vi "Crosswalk.vi"() -> ()   [LabVIEW 2020]
uses:
  Auto.ctl
  People.ctl
  State.ctl
panel:
  out "Time Elapsed (s)":u32
  in  "Button":bool
  in  "stop":bool
  out "State":T1
  out "Pedestrians":T2
  out "Vehicles":T3
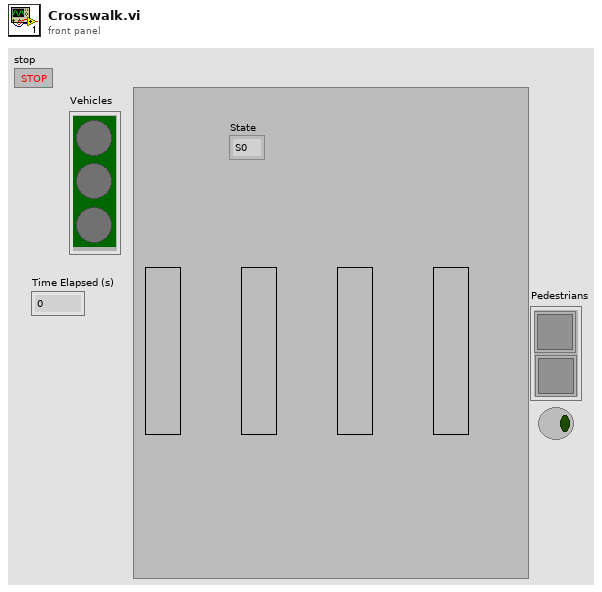
[diagram p1: front panel]
types:
  T1 = typedef "State.ctl" = enum16{"S0", "S1", "S2", "S3", "S4"}
  T2 = typedef "People.ctl" = cluster{"Red":bool, "Green":bool}
  T3 = typedef "Auto.ctl" = cluster{"Red":bool, "Yellow":bool, "Green":bool}
  T4 = enum8{"Enabled", "Disabled", "Disabled and Grayed Out"}
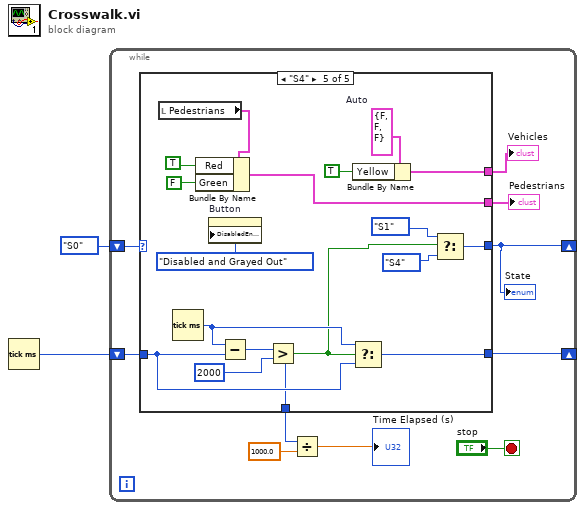
[diagram p0: block diagram]
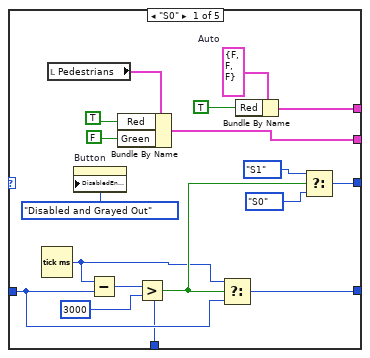
[diagram p2: hidden frame]
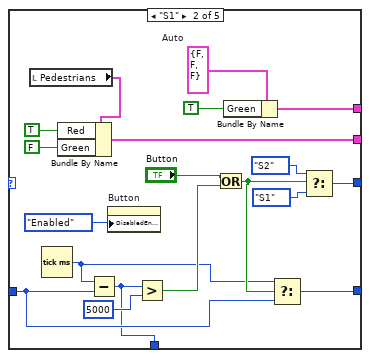
[diagram p3: hidden frame]
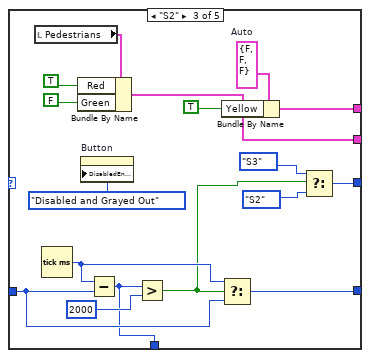
[diagram p4: hidden frame]
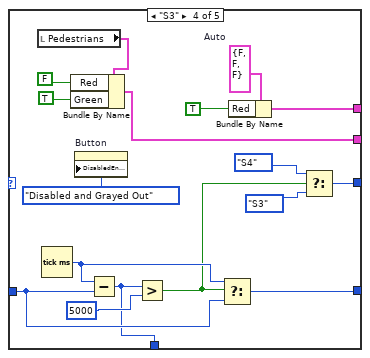
[diagram p5: hidden frame]
diagram:
  n1 = Tick Count (ms)() -> (millisecond timer value=w1:u32)
  n2 = while {
    shift-right: [w7] -> _
    shift-left: State."S0" ("Состояние") -> [w11]
    shift-right: [w10] -> _
    shift-left: w1 -> [w3]
    stop <- "stop" stop-if-true
    n3 = case shown="\"S4\"" w11 {
      tunnel: w3 -> [w27 w46 w62 w79 w96]
      tunnel: [w28 w47 w63 w80 w97] -> w10
      tunnel: [w24 w44 w60 w77 w94] -> w7
      tunnel: [w20 w38 w54 w71 w88] -> w9
      tunnel: [w17 w36 w52 w69 w86] -> w8
      tunnel: [w15 w32 w50 w67 w84] -> w5
      frame "S0" {
        w22 = T3 {"Red"=FALSE, "Yellow"=FALSE, "Green"=FALSE}  # Auto
        n4 = Tick Count (ms)() -> (millisecond timer value=w14:u32)
        n5 = local read "Pedestrians"() -> (w18:T2)
        n6 = property on="Button" class="Bool (strict)"("DisabledEnum"=T4."Disabled and Grayed Out" ("Disabled")) -> ()  [unwired: 2 in, 2 out]
        n7 = Subtract(x=w14, y=w27) -> (x-y=w15:u32)
        n8 = Bundle By Name(cluster=w18, "Red"=TRUE ("Красный"), "Green"=FALSE ("Зеленый")) -> (w17:T2)
        n9 = Greater?(x=w15, y=u32 3000) -> (0:w26:bool)
        n10 = Select(t=w14, s=w26, f=w27) -> (s? t:f=w28:u32)
        n11 = Bundle By Name(cluster=w22, "Red"=TRUE ("Красный")) -> (w20:T3)
        n12 = Select(t=State."S1" ("Состояние"), s=w26, f=State."S0" ("Состояние")) -> (s? t:f=w24:T1)
      }
      frame "S1" {
        w37 = T3 {"Red"=FALSE, "Yellow"=FALSE, "Green"=FALSE}  # Auto
        n13 = local read "Pedestrians"() -> (w40:T2)
        n14 = Tick Count (ms)() -> (millisecond timer value=w31:u32)
        n15 = Bundle By Name(cluster=w40, "Red"=TRUE ("Красный"), "Green"=FALSE ("Зеленый")) -> (w36:T2)
        n16 = Subtract(x=w31, y=w46) -> (x-y=w32:u32)
        n17 = property on="Button" class="Bool (strict)"("DisabledEnum"=T4."Enabled" ("Disabled")) -> ()  [unwired: 2 in, 2 out]
        n18 = Greater?(x=w32, y=u32 5000) -> (0:w35:bool)
        n19 = Or(x="Button", y=w35) -> (x .or. y?=w33:bool)
        n20 = Bundle By Name(cluster=w37, "Green"=TRUE ("Красный")) -> (w38:T3)
        n21 = Select(t=w31, s=w33, f=w46) -> (s? t:f=w47:u32)
        n22 = Select(t=State."S2" ("Состояние"), s=w33, f=State."S1" ("Состояние")) -> (s? t:f=w44:T1)
      }
      frame "S2" {
        w53 = T3 {"Red"=FALSE, "Yellow"=FALSE, "Green"=FALSE}  # Auto
        n23 = local read "Pedestrians"() -> (w56:T2)
        n24 = Tick Count (ms)() -> (millisecond timer value=w64:u32)
        n25 = Bundle By Name(cluster=w56, "Red"=TRUE ("Красный"), "Green"=FALSE ("Зеленый")) -> (w52:T2)
        n26 = property on="Button" class="Bool (strict)"("DisabledEnum"=T4."Disabled and Grayed Out" ("Disabled")) -> ()  [unwired: 2 in, 2 out]
        n27 = Subtract(x=w64, y=w62) -> (x-y=w50:u32)
        n28 = Greater?(x=w50, y=u32 2000) -> (0:w51:bool)
        n29 = Bundle By Name(cluster=w53, "Yellow"=TRUE ("Красный")) -> (w54:T3)
        n30 = Select(t=w64, s=w51, f=w62) -> (s? t:f=w63:u32)
        n31 = Select(t=State."S3" ("Состояние"), s=w51, f=State."S2" ("Состояние")) -> (s? t:f=w60:T1)
      }
      frame "S3" {
        w70 = T3 {"Red"=FALSE, "Yellow"=FALSE, "Green"=FALSE}  # Auto
        n32 = local read "Pedestrians"() -> (w73:T2)
        n33 = Tick Count (ms)() -> (millisecond timer value=w81:u32)
        n34 = Bundle By Name(cluster=w73, "Red"=FALSE ("Красный"), "Green"=TRUE ("Зеленый")) -> (w69:T2)
        n35 = property on="Button" class="Bool (strict)"("DisabledEnum"=T4."Disabled and Grayed Out" ("Disabled")) -> ()  [unwired: 2 in, 2 out]
        n36 = Subtract(x=w81, y=w79) -> (x-y=w67:u32)
        n37 = Greater?(x=w67, y=u32 5000) -> (0:w68:bool)
        n38 = Select(t=w81, s=w68, f=w79) -> (s? t:f=w80:u32)
        n39 = Bundle By Name(cluster=w70, "Red"=TRUE ("Красный")) -> (w71:T3)
        n40 = Select(t=State."S4" ("Состояние"), s=w68, f=State."S3" ("Состояние")) -> (s? t:f=w77:T1)
      }
      frame "S4" {
        w87 = T3 {"Red"=FALSE, "Yellow"=FALSE, "Green"=FALSE}  # Auto
        n41 = local read "Pedestrians"() -> (w90:T2)
        n42 = Tick Count (ms)() -> (millisecond timer value=w98:u32)
        n43 = Bundle By Name(cluster=w90, "Red"=TRUE ("Красный"), "Green"=FALSE ("Зеленый")) -> (w86:T2)
        n44 = property on="Button" class="Bool (strict)"("DisabledEnum"=T4."Disabled and Grayed Out" ("Disabled")) -> ()  [unwired: 2 in, 2 out]
        n45 = Subtract(x=w98, y=w96) -> (x-y=w84:u32)
        n46 = Greater?(x=w84, y=u32 2000) -> (0:w85:bool)
        n47 = Bundle By Name(cluster=w87, "Yellow"=TRUE ("Красный")) -> (w88:T3)
        n48 = Select(t=w98, s=w85, f=w96) -> (s? t:f=w97:u32)
        n49 = Select(t=State."S1" ("Состояние"), s=w85, f=State."S4" ("Состояние")) -> (s? t:f=w94:T1)
      }
    }
    "Vehicles" <- w9
    "Pedestrians" <- w8
    "State" <- w7
    n50 = Divide(x=w5, y=1000.0) -> (x/y=→"Time Elapsed (s)":dbl)
  }
